vi "System Error Logging.vi"(8 "error in":errorcluster, 11 "Error Clear":bool) -> (0 "error out":errorcluster)   [LabVIEW 2023, in "GUI.lvlib"]
uses:
  GUI.lvlib
  Control/SystemLog.ctl
  HardwareAbstractionLayer_LVOOP/Database/Database.lvclass
  <userlib>/_OpenG.lib/appcontrol/appcontrol.llb/openg_application_control.lvlib
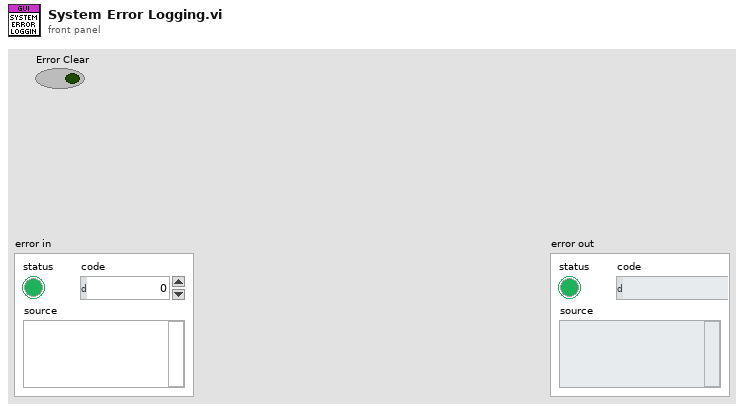
[diagram p1: front panel]
types:
  T1 = typedef "GUI.lvlib/SystemLog.ctl" = cluster{"VI_NAME":string, "ERROR_MESSAGE":string}
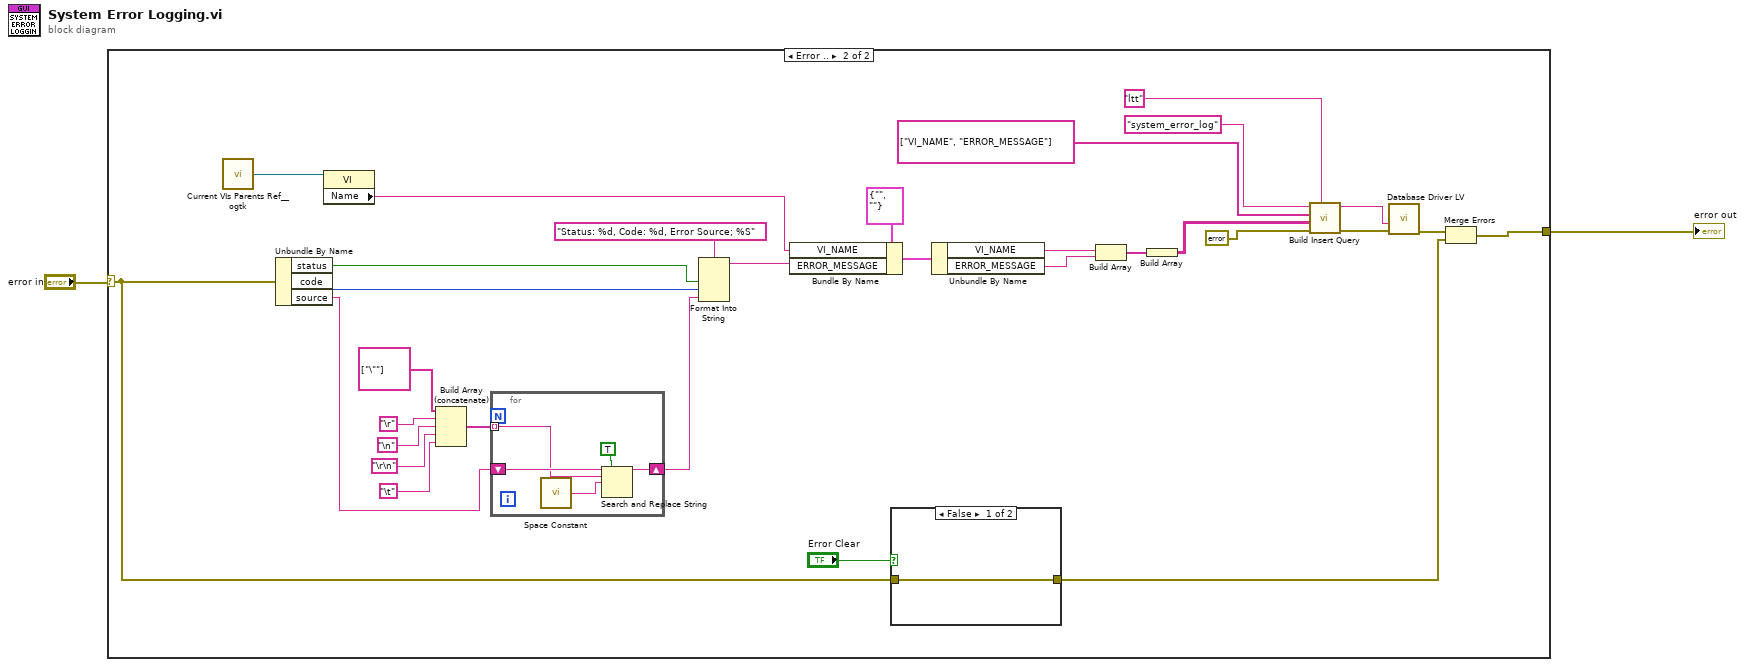
[diagram p0: block diagram]
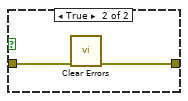
[diagram p3: hidden frame]
diagram:
  n1 = case shown="Error .." "error in" {
    selector: "error in" -> [w3 w14]
    tunnel: [w3 w15] -> w1
    frame No Error {
    }
    frame Error {
      n2 = call <userlib>:"Current VIs Parents Ref__ogtk.vi"() -> ("Calling VI's Reference"=w23:refnum<vi>)  [unwired: 2 in]
      n3 = Unbundle By Name(w14) -> ("status"=w33:bool, "code"=w32:i32, "source"=w5:string)
      n4 = property class="VI"(reference=w23) -> ("Name"=w22:string)  [unwired: 1 in, 2 out]
      n5 = Build Array (concatenate)(string[] ["\""], "\r", "\n", "\r\n", "\t") -> (w11:string[])
      n6 = for {
        tunnel: w11 -> [w36] mode=indexing
        shift-right: [w37] -> w4
        shift-left: w5 -> [w38]
        n7 = call <vilib>:"Space Constant.vi"() -> ("String"=w35:string)
        n8 = Search and Replace String(replace all?=TRUE ("replace all? (F)"), input string=w38, search string=w36, replace string=w35) -> (result string=w37:string)  [unwired: 4 in, 3 out]
      }
      n9 = Format Into String(format string="Status: %d, Code: %d, Error Source; %S", w33, w32, w4) -> (resulting string=w30:string)  [unwired: 2 in, 1 out]
      n10 = Bundle By Name(cluster=T1 {"VI_NAME"="", "ERROR_MESSAGE"=""} ("SystemLog"), "VI_NAME"=w22, "ERROR_MESSAGE"=w30) -> (w26:T1)
      n11 = case shown="False" "Error Clear" {
        tunnel: w14 -> [w40 w42]
        tunnel: [w40 w41] -> w13
        frame False {
        }
        frame True {
          n12 = call <vilib>:"Clear Errors.vi"("error in (no error)"=w42) -> ("error out"=w41:errorcluster)  [unwired: 5 in, 1 out]
        }
      }
      n13 = Unbundle By Name(w26) -> ("VI_NAME"=w25:string, "ERROR_MESSAGE"=w24:string)
      n14 = Build Array(w25, w24) -> (w20:string[])
      n15 = Build Array(w20) -> (w19:string[][])
      n16 = call "Build Insert Query.vi"("Schema Name"="ltt", "error in (no error)"=errorcluster {"status"=FALSE, "code"=0, "source"=""}, "Data"=w19, "Column Names"=string[] ["VI_NAME", "ERROR_MESSAGE"], "Table Name"="system_error_log") -> ("error out"=w21:errorcluster, "SQL"=w16:string)  [unwired: 5 in]
      n17 = call "Database Driver LV.vi"("error in"=w21, "SQL query"=w16) -> ("error out"=w17:errorcluster)  [unwired: 6 in, 3 out]
      n18 = Merge Errors(w17, w13) -> (w15:errorcluster)
    }
  }
  "error out" <- w1
